vi "FTW-SQLite-Core-Construct.vi"(0 "Database URI":string, 2 "Database Type":T1, 5 "Access Mode":T2, 11 "error in":errorcluster) -> (4 "SQLite Connection":refnum<data-value>, 6 "SQLite Version":string, 15 "error out":errorcluster)   [LabVIEW 2014]
uses:
  FTW-SQLite-Core-AccessMode.ctl
  FTW-SQLite-Core-DatabaseType.ctl
  FTW-SQLite-Core-Structure.ctl
panel:
  # "Inputs"
  # "Outputs"
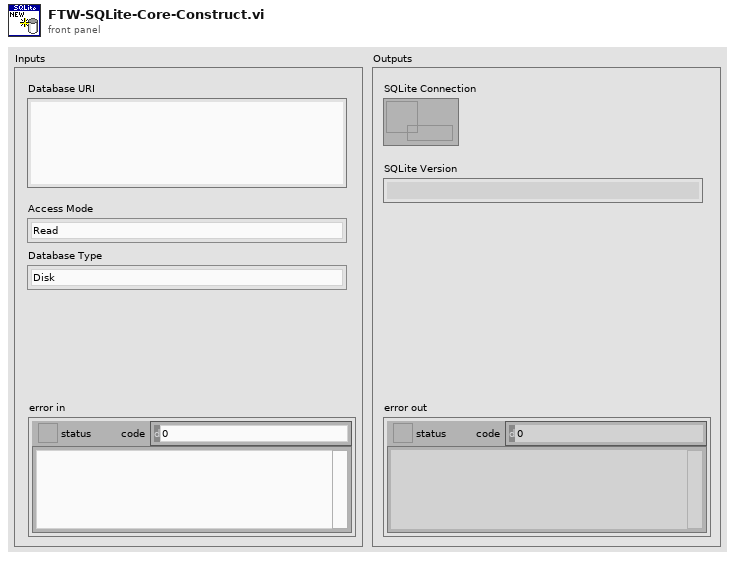
[diagram p1: front panel]
types:
  T1 = typedef "FTW-SQLite-Core-DatabaseType.ctl" = enum16{"Disk", "Memory"}
  T2 = typedef "FTW-SQLite-Core-AccessMode.ctl" = enum16{"Read", "Read/Write", "Read/Write/Create"}
  T3 = typedef "FTW-SQLite-Core-Structure.ctl" = cluster{"Connection":u64}
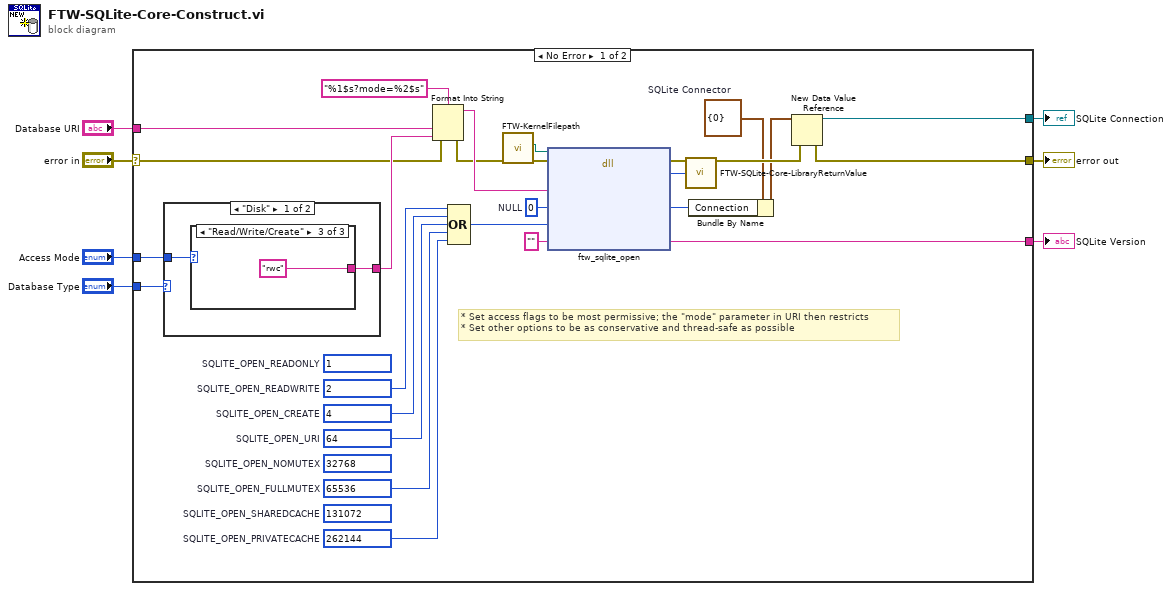
[diagram p0: block diagram]
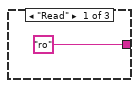
[diagram p2: hidden frame]
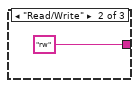
[diagram p3: hidden frame]
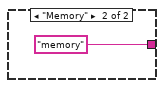
[diagram p4: hidden frame]
diagram:
  n1 = case shown="No Error" "error in" {
    selector: "error in" -> [w28 w41]
    tunnel: [w16 w41] -> w7
    tunnel: [w15 _] -> w1
    tunnel: [w11 _] -> w5
    tunnel: "Database URI" -> [w31 _]
    tunnel: "Access Mode" -> [w33 _]
    tunnel: "Database Type" -> [w22 _]
    frame No Error {
      w14 = T3 {"Connection"=0}  # SQLite Connector
      w18 = u64 0  # NULL
      w23 = u32 262144  # SQLITE_OPEN_PRIVATECACHE
      (unwired) u32 131072  # SQLITE_OPEN_SHAREDCACHE
      w24 = u32 65536  # SQLITE_OPEN_FULLMUTEX
      (unwired) u32 32768  # SQLITE_OPEN_NOMUTEX
      w25 = u32 64  # SQLITE_OPEN_URI
      w26 = u32 4  # SQLITE_OPEN_CREATE
      w27 = u32 2  # SQLITE_OPEN_READWRITE
      (unwired) u32 1  # SQLITE_OPEN_READONLY
      # "* Set access flags to be most permissive; the \"mode\" parameter in URI then restricts\n* Set other options to be as conservative and thread-safe as possible"
      n2 = case shown="\"Disk\"" w22 {
        tunnel: w33 -> [w36 _]
        tunnel: [w35 "memory"] -> w30
        frame "Disk" {
          n3 = case shown="\"Read/Write/Create\"" w36 {
            tunnel: ["ro" "rw" "rwc"] -> w35
            frame "Read" {
            }
            frame "Read/Write" {
            }
            frame "Read/Write/Create" {
            }
          }
        }
        frame "Memory" {
        }
      }
      n4 = Format Into String(format string="%1$s?mode=%2$s", error in=w28, w31, w30) -> (resulting string=w13:string, error out=w10:errorcluster)  [unwired: 1 in]
      n5 = Compound Arithmetic op=OR(w27, w26, w25, w24, w23) -> (w29:u32)
      n6 = call "FTW-KernelFilepath.vi"("error in"=w10) -> ("error out"=w8:errorcluster, "Library Filepath"=w9:path)  [unwired: 8 in, 1 out]
      n7 = dll-call lib="?" fn="ftw_sqlite_open"(path in=w9, error in=w8, "Database URI"=w13, "Connection Handle"=w18, "Flags"=w29, "Library Version"="") -> (error out=w21:errorcluster, "Return Value"=w20:i32, "Connection Handle"=w19:u64, "Library Version"=w11:string)  [unwired: 3 in, 1 out]
      n8 = call "FTW-SQLite-Core-LibraryReturnValue.vi"("error in"=w21, "Return Value"=w20) -> ("error out"=w34:errorcluster)  [unwired: 13 in]
      n9 = Bundle By Name(cluster=w14, "Connection"=w19) -> (w17:T3)
      n10 = New Data Value Reference(data value=w17, error in=w34) -> (data value reference=w15:refnum<data-value>, error out=w16:errorcluster)
    }
    frame Error {
    }
  }
  "error out" <- w7
  "SQLite Version" <- w5
  "SQLite Connection" <- w1
